vi "_GroupCommandInOut.vi"(2 "error in":errorcluster, 3 "args_in":cluster{"num data":u8[], "str data":string[]}[](array[cluster]), 4 "command_name":string, 5 "group id":i32) -> (0 "error out":errorcluster, 1 "args_out":cluster{"num data":u8[], "str data":string[]}[](array[cluster]))   [LabVIEW 2014, in "tango.lvlib"]
uses:
  tango.lvlib
  tango_binding.so
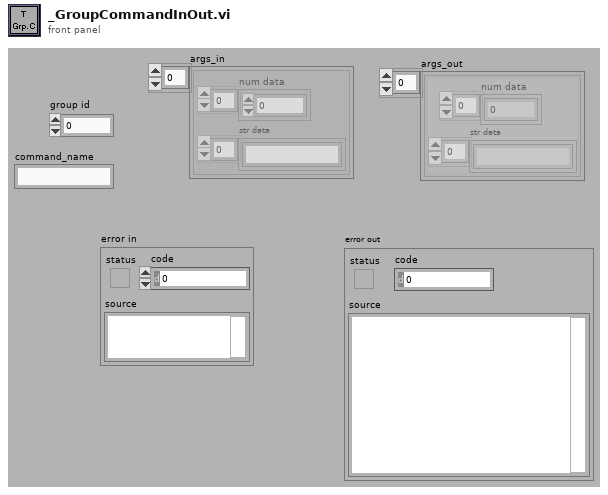
[diagram p1: front panel]
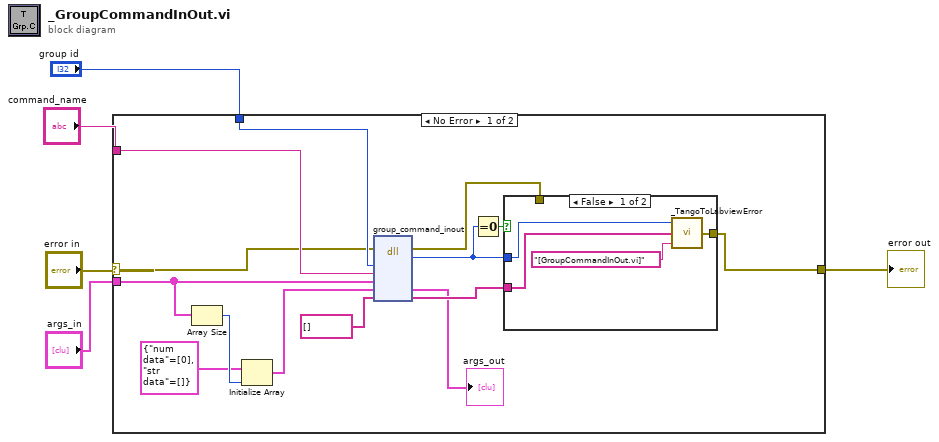
[diagram p0: block diagram]
diagram:
  n1 = case shown="No Error" "error in" {
    selector: "error in" -> [w12 w25]
    tunnel: [w17 w25] -> w4
    tunnel: "command_name" -> [w15 _]
    tunnel: "group id" -> [w14 _]
    tunnel: "args_in" -> [w11 _]
    frame No Error {
      n2 = Array Size(array=w11) -> (size(s)=w10:i32)
      n3 = Initialize Array(cluster{"num data":u8[], "str data":string[]} {"num data"=[0], "str data"=[]} ("ArgIO"), w10) -> (w9:cluster{"num data":u8[], "str data":string[]}[])
      n4 = dll-call lib="tango_binding.*" fn="group_command_inout"(error in=w12, "group_id"=w14, "command_name"=w15, "args_in"=w11, "args_out"=w9, "error_stack"=string[] [] ("error stack")) -> (error out=w13:errorcluster, "type de retour"=w16:i32, "args_out"=→"args_out":cluster{"num data":u8[], "str data":string[]}[], "error_stack"=w18:string[])  [unwired: 5 in, 1 out]
      n5 = Equal To 0?(x=w16) -> (x = 0?=w19:bool)
      n6 = case shown="False" w19 {
        tunnel: [w20 w24] -> w17
        tunnel: w16 -> [w22 _]
        tunnel: w18 -> [w21 _]
        tunnel: w13 -> [_ w24]
        frame False {
          n7 = call "_TangoToLabviewError.vi"("location"="[GroupCommandInOut.vi]", "error stack"=w21, "error code"=w22) -> ("error out"=w20:errorcluster)
        }
        frame True {
        }
      }
    }
    frame Error {
    }
  }
  "error out" <- w4
